vi "Main Page.vi"(8 "error in (no error)":errorcluster, 11 "Node Ptr":T1 format="%.0x") -> (0 "error out":errorcluster)   [LabVIEW 2026, in "WebPage Addon System Explorer.lvlib"]
uses:
  WebPage Addon System Explorer.lvlib
  <vilib>/NI VeriStand/Custom Device API/Custom Device Item Ref.ctl
  <vilib>/NI VeriStand/Custom Device API/Get Item Property (Double).vi
  <vilib>/NI VeriStand/Custom Device API/Get Item Property (U32).vi
  <vilib>/NI VeriStand/Custom Device API/Get Item Property (String).vi
  <vilib>/NI VeriStand/Custom Device API/Set Item Property (Double).vi
  <vilib>/NI VeriStand/Custom Device API/Set Item Property (String).vi
  <vilib>/NI VeriStand/Custom Device API/Set Item Property (U32).vi
  <vilib>/NI VeriStand/Custom Device API/Custom Device API.lvlib
panel:
  in  "gRPC Port":u32=53251
  in  "Hosted Port":u32=8382
  in  "Hosted IP Address":string
  out "Published Channels":string[][](table)
  in  "Update Rate (Hz)":dbl=1.0 min=0.5 max=100.0 step=0.5
  out "Version":string
  in  "SHDocVw.IWebBrowser":refnum<k7>(container)
  in  "Specific Header":cluster{"Section Name":string}={"Section Name"="Custom Device Item Settings"}
  in  "General Header":cluster{"Section Name":string}={"Section Name"="General Custom Device Settings"}
  in  "Name":string
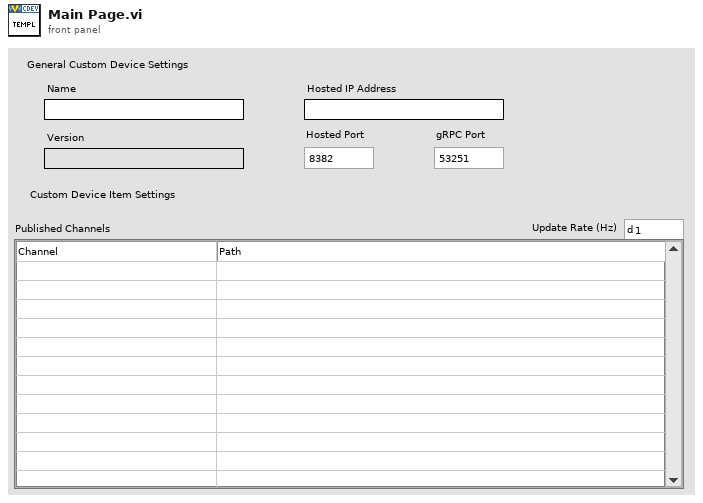
[diagram p1: front panel]
types:
  T1 = typedef "Custom Device API.lvlib/Custom Device Item Ref.ctl" = u64
  T2 = typedef "Custom Device API.lvlib/Custom Device Item Info.ctl" = cluster{"Name":string, "Is Channel":bool, "GUID":string, "Is Waveform":bool}
  T3 = typedef "Custom Device API.lvlib/Custom Device Pointer.ctl" = refnum<k24>
  T4 = typedef "Custom Device API.lvlib/Custom Device Commands.ctl" = enum16{"Default", "Item renamed", "Shutdown", "Dynamic button pressed"}
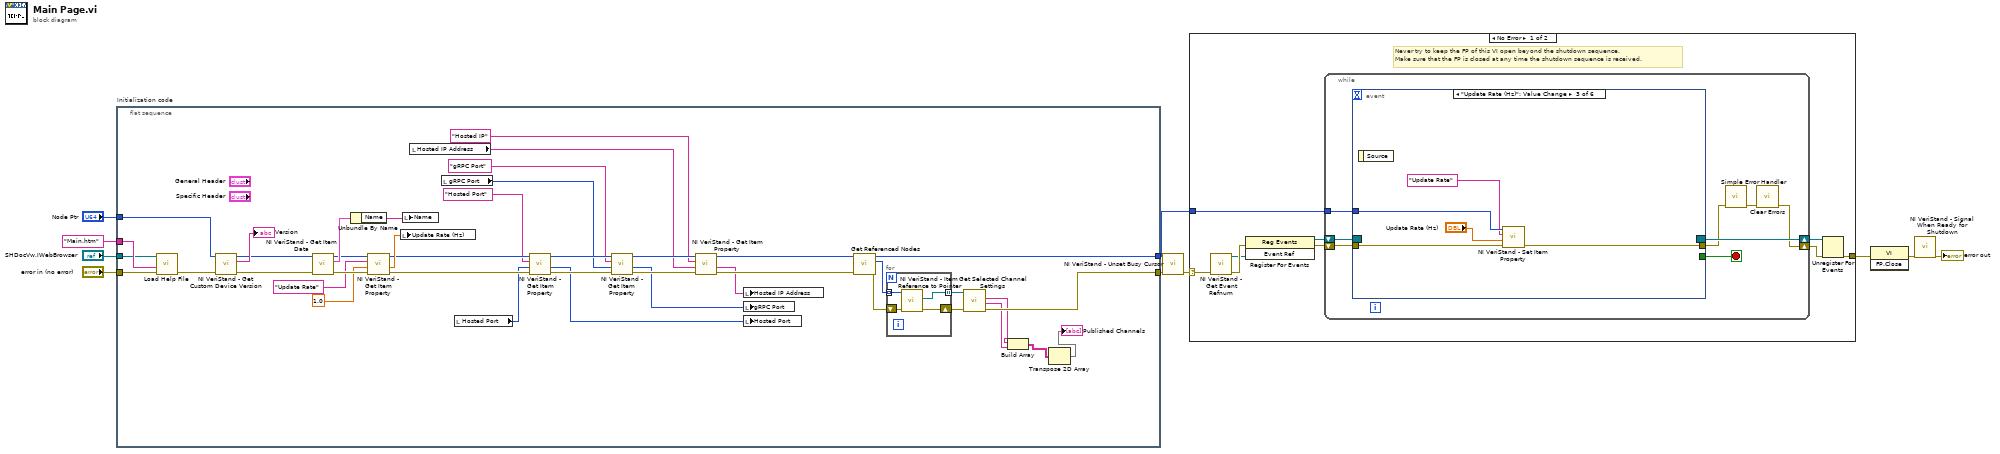
[diagram p0: block diagram]
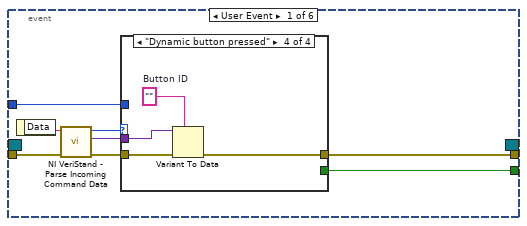
[diagram p2: hidden frame]
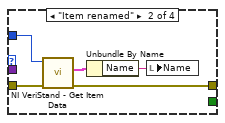
[diagram p4: hidden frame]
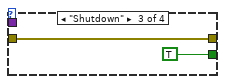
[diagram p5: hidden frame]
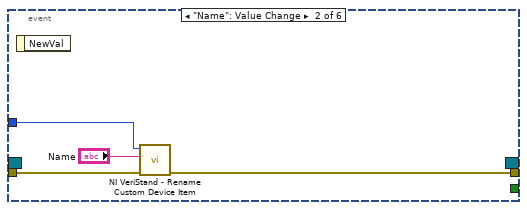
[diagram p6: hidden frame]
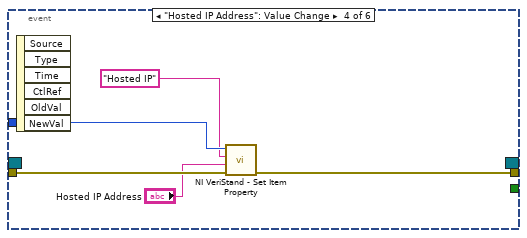
[diagram p7: hidden frame]
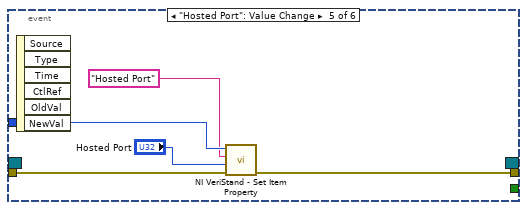
[diagram p8: hidden frame]
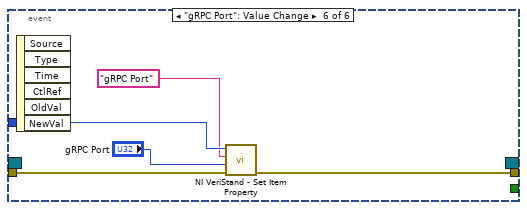
[diagram p9: hidden frame]
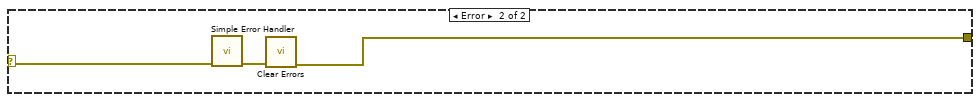
[diagram p10: hidden frame]
diagram:
  n1 = flat-sequence "Initialization code" {
    tunnel: "error in (no error)" -> [w48]
    tunnel: "Node Ptr" -> [w51]
    tunnel: [w36] -> w6
    tunnel: [w39] -> w3
    tunnel: "SHDocVw.IWebBrowser" -> [w45]
    tunnel: "Main.htm" ("HTML File") -> [w46]
    frame #0 {
      n2 = call "Load Help File.vi"("error in (no error)"=w48, "HTML File to Load"=w46, "Browser"=w45) -> ("error out"=w47:errorcluster)  [unwired: 8 in]
      n3 = call <vilib>:"NI VeriStand - Get Custom Device Version.vi"("error in (no error)"=w47, "Device Ref in"=w51) -> ("error out"=w29:errorcluster, "Value"=→"Version":string, "Device Ref out"=w28:T1)  [unwired: 7 in]
      n4 = call <vilib>:"NI VeriStand - Get Item Data.vi"("error in (no error)"=w29, "Item Ref in"=w28) -> ("error out"=w44:errorcluster, "Item Info"=w52:T2, "Item Ref out"=w43:T1)  [unwired: 7 out]
      n5 = Unbundle By Name(w52) -> ("Name"=w49:string)
      n6 = call-poly <vilib>:"NI VeriStand - Get Item Property.vi"("error in (no error)"=w44, "Default Value"=1.0, "Property Name"="Update Rate", "Item Ref in"=w43) -> ("error out"=w27:errorcluster, "Value"=w41:dbl, "Item Ref out"=w26:T1)  [unwired: 4 in, 1 out]
      n7 = local write "Update Rate (Hz)"(w41) -> ()
      n8 = local write "Name"(w49) -> ()
      n9 = local read "Hosted IP Address"() -> (w13:string)
      n10 = local read "gRPC Port"() -> (w11:u32)
      n11 = local read "Hosted Port"() -> (w12:u32)
      n12 = call-poly <vilib>:"NI VeriStand - Get Item Property.vi"("error in (no error)"=w27, "Default Value"=w12, "Property Name"="Hosted Port", "Item Ref in"=w26) -> ("error out"=w23:errorcluster, "Value"=w17:u32, "Item Ref out"=w25:T1)  [unwired: 4 in, 1 out]
      n13 = call-poly <vilib>:"NI VeriStand - Get Item Property.vi"("error in (no error)"=w23, "Default Value"=w11, "Property Name"="gRPC Port", "Item Ref in"=w25) -> ("error out"=w22:errorcluster, "Value"=w16:u32, "Item Ref out"=w24:T1)  [unwired: 4 in, 1 out]
      n14 = call-poly <vilib>:"NI VeriStand - Get Item Property.vi"("error in (no error)"=w22, "Default Value"=w13, "Property Name"="Hosted IP", "Item Ref in"=w24) -> ("error out"=w21:errorcluster, "Value"=w15:string, "Item Ref out"=w14:T1)  [unwired: 4 in, 1 out]
      n15 = local write "Hosted IP Address"(w15) -> ()
      n16 = local write "gRPC Port"(w16) -> ()
      n17 = local write "Hosted Port"(w17) -> ()
      n18 = call "Get Referenced Nodes.vi"("error in (no error)"=w21, "Item Ref in"=w14) -> ("error out"=w38:errorcluster, "Array"=w35:T1[], "Item Ref out"=w39:T1)  [unwired: 7 in]
      n19 = for {
        shift-right: [w55] -> w37
        shift-left: w38 -> [w56]
        tunnel: w35 -> [w54] mode=indexing
        tunnel: [w53] -> w34 mode=indexing
        n20 = call <vilib>:"NI VeriStand - Item Reference to Pointer.vi"("error in (no error)"=w56, "Item Ref in"=w54) -> ("error out"=w55:errorcluster, "Node Pointer"=w53:T3)  [unwired: 6 in, 2 out]
      }
      n21 = call "Get Selected Channel Settings.vi"("error in (no error)"=w37, "GetCheckBoxSelections"=w34) -> ("error out"=w36:errorcluster, "Path"=w32:string[], "Name"=w33:string[])  [unwired: 6 in, 1 out]
      n22 = Build Array(w33, w32) -> (w31:string[][])
      n23 = Transpose 2D Array(2D array=w31) -> (transposed array=→"Published Channels":string[][])
    }
  }
  n24 = call <vilib>:"NI VeriStand - Unset Busy Cursor.vi"("error in (no error)"=w6) -> ("error out"=w5:errorcluster)  [unwired: 10 out]
  n25 = case shown="No Error" w5 {
    selector: w5 -> [w57 w120]
    tunnel: [w62 w118] -> w10
    tunnel: w3 -> [w58 _]
    frame No Error {
      # "Never try to keep the FP of this VI open beyond the shutdown sequence.\nMake sure that the FP is closed at any time the shutdown sequence is received."
      n26 = call <vilib>:"NI VeriStand - Get Event Refnum.vi"("error in (no error)"=w57) -> ("error out"=w65:errorcluster, "Event Ref"=w61:refnum<user-event>)  [unwired: 9 out]
      n27 = register-events(error in=w65, w61) -> (reference out=w59:refnum<event-registration>, error out=w60:errorcluster)  [unwired: 1 in]
      n28 = while {
        tunnel: w58 -> [w69]
        shift-right: [w66] -> w63
        shift-left: w60 -> [w72]
        shift-right: [w73] -> w64
        shift-left: w59 -> [w71]
        stop <- w70 stop-if-true
        n29 = event shown="[2] \"Update Rate (Hz)\": Value Change" {
          selector: w71 -> [_ _ _ _ _ _]
          dyn-events: [_ _ _ _ _ _] -> w73
          timeout: _ -> [_ _ _ _ _ _]
          tunnel: w72 -> [w81 w97 w102 w107 w112 w117]
          tunnel: [w77 _ _ _ _ _] -> w70
          tunnel: [w76 w96 w100 w105 w110 w115] -> w68
          tunnel: w69 -> [w75 w95 w101 w106 w111 w116]
          event User Event {
            n30 = event-data() -> ("Data"=w80:string)  [unwired: 1 out]
            n31 = call <vilib>:"NI VeriStand - Parse Incoming Command Data.vi"("error in (no error)"=w81, "Incoming data"=w80) -> ("error out"=w79:errorcluster, "Outgoing data"=w74:variant, "Action"=w78:T4)  [unwired: 7 out]
            n32 = case shown="\"Dynamic button pressed\"" w78 {
              tunnel: w79 -> [w82 w87 w88 w93]
              tunnel: [_ _ TRUE _] -> w77
              tunnel: [w82 w84 w88 w90] -> w76
              tunnel: w75 -> [_ w86 _ _]
              tunnel: w74 -> [_ _ _ w92]
              frame "Default", Default {
              }
              frame "Item renamed" {
                n33 = call <vilib>:"NI VeriStand - Get Item Data.vi"("error in (no error)"=w87, "Item Ref in"=w86) -> ("error out"=w84:errorcluster, "Item Info"=w85:T2)  [unwired: 8 out]
                n34 = Unbundle By Name(w85) -> ("Name"=w83:string)
                n35 = local write "Name"(w83) -> ()
              }
              frame "Shutdown" {
              }
              frame "Dynamic button pressed" {
                w91 = ""  # Button ID
                n36 = Variant To Data(error in=w93, type=w91, Variant=w92) -> (error out=w90:errorcluster)  [unwired: 1 out]
              }
            }
          }
          event "Name": Value Change {
            n37 = event-data() -> ()  [unwired: 2 out]
            n38 = call <vilib>:"NI VeriStand - Rename Custom Device Item.vi"("error in (no error)"=w97, "New Name"="Name", "Item Ref in"=w95) -> ("error out"=w96:errorcluster)  [unwired: 1 in, 7 out]
          }
          event "Update Rate (Hz)": Value Change {
            n39 = event-data() -> ()  [unwired: 2 out]
            n40 = call-poly <vilib>:"NI VeriStand - Set Item Property.vi"("error in (no error)"=w102, "Value"="Update Rate (Hz)", "Property Name"="Update Rate", "Item Ref in"=w101) -> ("error out"=w100:errorcluster)  [unwired: 5 in, 2 out]
          }
          event "Hosted IP Address": Value Change {
            n41 = event-data() -> ()  [unwired: 7 out]
            n42 = call-poly <vilib>:"NI VeriStand - Set Item Property.vi"("error in (no error)"=w107, "Value"="Hosted IP Address", "Property Name"="Hosted IP", "Item Ref in"=w106) -> ("error out"=w105:errorcluster)  [unwired: 5 in, 2 out]
          }
          event "Hosted Port": Value Change {
            n43 = event-data() -> ()  [unwired: 7 out]
            n44 = call-poly <vilib>:"NI VeriStand - Set Item Property.vi"("error in (no error)"=w112, "Value"="Hosted Port", "Property Name"="Hosted Port", "Item Ref in"=w111) -> ("error out"=w110:errorcluster)  [unwired: 5 in, 2 out]
          }
          event "gRPC Port": Value Change {
            n45 = event-data() -> ()  [unwired: 7 out]
            n46 = call-poly <vilib>:"NI VeriStand - Set Item Property.vi"("error in (no error)"=w117, "Value"="gRPC Port", "Property Name"="gRPC Port", "Item Ref in"=w116) -> ("error out"=w115:errorcluster)  [unwired: 5 in, 2 out]
          }
        }
        n47 = call <vilib>:"Simple Error Handler.vi"("error in (no error)"=w68) -> ("error out"=w67:errorcluster)  [unwired: 1 in, 7 out]
        n48 = call <vilib>:"Clear Errors.vi"("error in (no error)"=w67) -> ("error out"=w66:errorcluster)  [unwired: 1 in, 5 out]
      }
      n49 = Unregister For Events(event registration refnum=w64, error in=w63) -> (error out=w62:errorcluster)
    }
    frame Error {
      n50 = call <vilib>:"Simple Error Handler.vi"("error in (no error)"=w120) -> ("error out"=w119:errorcluster)  [unwired: 1 in, 7 out]
      n51 = call <vilib>:"Clear Errors.vi"("error in (no error)"=w119) -> ("error out"=w118:errorcluster)  [unwired: 1 in, 5 out]
    }
  }
  n52 = invoke class="VI" method="FP.Close"(error in=w10) -> (error out=w9:errorcluster)  [unwired: 2 in, 2 out]
  n53 = call <vilib>:"NI VeriStand - Signal When Ready for Shutdown.vi"("error in (no error)"=w9) -> ("error out"=→"error out":errorcluster)  [unwired: 10 out]
